vi "CRYSet Graph Property.vi"(4 "PreviewGraph Ref":refnum<vi>, 6 "Splitters":refnum<vi>[](array[refnum]), 7 "pGraph VI In":refnum<vi>, 8 "Panes":refnum<vi>[](array[refnum]), 9 "Graph Ref":refnum<vi>, 10 "Graph Type":string, 11 "Event Name":string) -> ()   [LabVIEW 2013]
uses:
  Control/CRYPolar Property.ctl
panel:
  in  "Polar Property":T1={"polar attributes"={"maximum"=2.0, "minimum"=0.0, "clip to min"=FALSE, "log"=FALSE, "grid color"=3381657, "plot color"=16711680, "fmt and prec"={"format"=enum."Decimal", "precision"=2}, "visible section"=4}, "Auto/Manual"=0, "Zero Adjust (deg)"=0, "Angle Increment (deg)"=0, "Mirror"=FALSE, "Auto Increment"=FALSE, "Total Rotatin (deg)"=0, "Discrete/Rannge"=0, "Show Name"=FALSE, "CurValues"=[], "CurIndex"=0, "CurColors"=[], "CurColors_Range"=[], "CurValues_Range"=[], "Pen"={"Width"=1, "Style"=enum."Solid"}, "BackgroundColor"=0} {"polar attributes"."minimum" format="%0.2f"; "polar attributes"."maximum" format="%0.2f"}
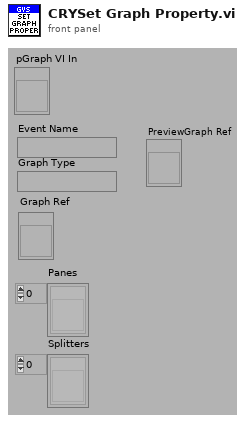
[diagram p1: front panel]
types:
  T1 = typedef "CRYPolar Property.ctl" = cluster{"polar attributes":cluster{"maximum":dbl, "minimum":dbl, "clip to min":bool, "log":bool, "grid color":u32, "plot color":u32, "fmt and prec":cluster{"format":enum8{"Decimal", "Scientific", "Engineering", "Binary", "Octal", "Hex"}, "precision":u8}, "visible section":u16}, "Auto/Manual":u16, "Zero Adjust (deg)":i32, "Angle Increment (deg)":i32, "Mirror":bool, "Auto Increment":bool, "Total Rotatin (deg)":i32, "Discrete/Rannge":u16, "Show Name":bool, "CurValues":dbl[], "CurIndex":u16, "CurColors":u32[], "CurColors_Range":u32[], "CurValues_Range":dbl[], "Pen":cluster{"Width":u16, "Style":enum32{"Solid", "Dash", "Dot", "DashDot", "DashDotDot"}}, "BackgroundColor":u32}
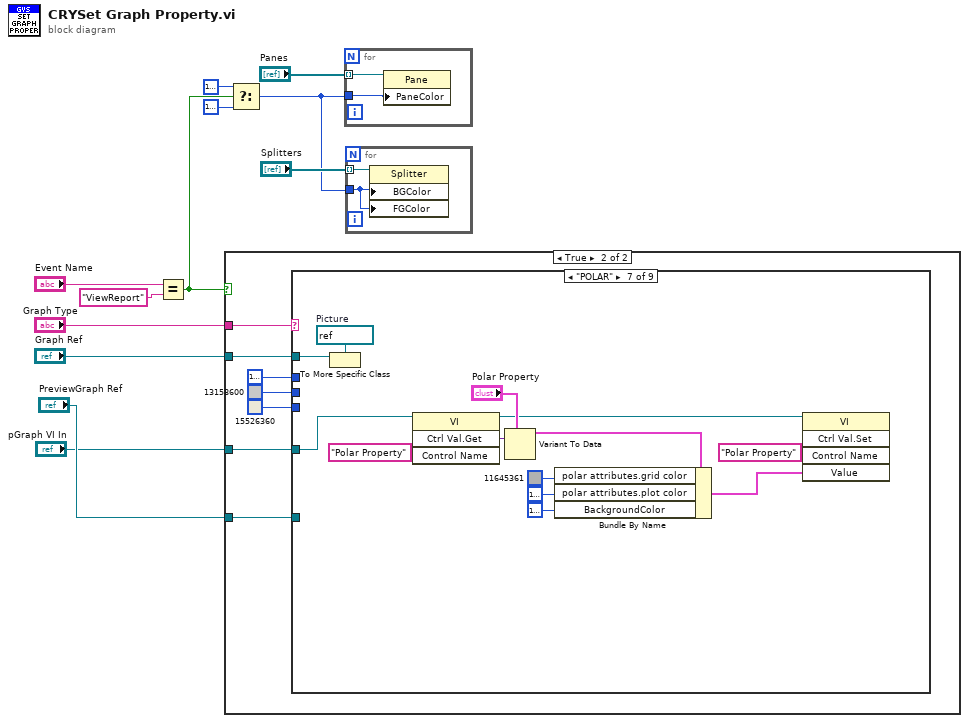
[diagram p0: block diagram]
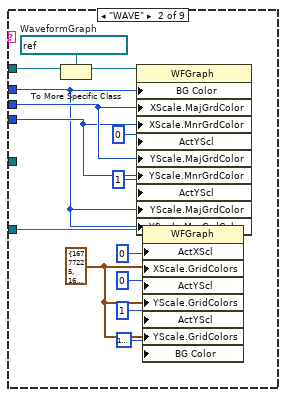
[diagram p4: hidden frame]
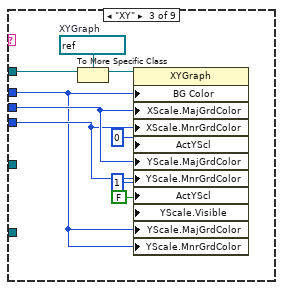
[diagram p5: hidden frame]
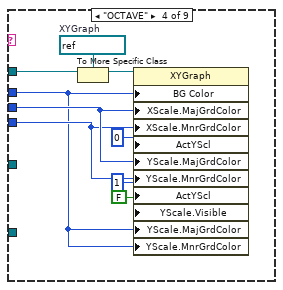
[diagram p6: hidden frame]
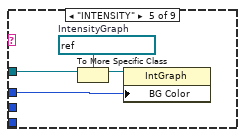
[diagram p7: hidden frame]
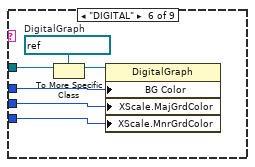
[diagram p8: hidden frame]
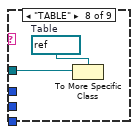
[diagram p9: hidden frame]
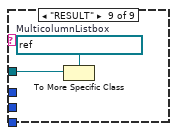
[diagram p10: hidden frame]
diagram:
  n1 = Equal?(x="Event Name", y="ViewReport" ("regular expression")) -> (x = y?=w5:bool)
  n2 = case shown="True" w5 {
    tunnel: "Graph Type" -> [_ w19]
    tunnel: "Graph Ref" -> [_ w18]
    tunnel: "PreviewGraph Ref" -> [_ w14]
    tunnel: "pGraph VI In" -> [_ w13]
    frame False {
    }
    frame True {
      n3 = case shown="\"POLAR\"" w19 {
        tunnel: w18 -> [_ w29 w38 w47 w55 w58 w74 w76 w78]
        tunnel: u32 16777226 -> [_ w26 w34 w43 w52 w61 _ _ _]
        tunnel: u32 13158600 -> [_ w31 w40 w49 _ w60 _ _ _]
        tunnel: u32 15526360 -> [_ w30 w39 w48 _ w59 _ _ _]
        tunnel: w14 -> [_ w22 _ _ _ _ _ _ _]
        tunnel: w13 -> [_ _ _ _ _ _ w69 _ _]
        frame Default {
        }
        frame "WAVE" {
          w23 = cluster{u32, u32} {16777225, 16777225}
          w27 = refnum<vi> refnum  # WaveformGraph
          n4 = To More Specific Class(target class=w27, reference=w29) -> (specific class reference=w28:refnum<vi>)  [unwired: 1 in, 1 out]
          n5 = property class="WFGraph"(reference=w28, "BG Color"=w26, "XScale.MajGrdColor"=w31, "XScale.MnrGrdColor"=w30, "ActYScl"=0 ("Active Y Scale"), "YScale.MajGrdColor"=w31, "YScale.MnrGrdColor"=w30, "ActYScl"=1 ("Active Y Scale"), "YScale.MajGrdColor"=w26, "YScale.MnrGrdColor"=w26) -> ()  [unwired: 1 in, 2 out]
          n6 = property on="Property Node" class="WFGraph"(reference=w22, "ActXScl"=0 ("Active X Scale"), "XScale.GridColors"=w23, "ActYScl"=0 ("Active Y Scale"), "YScale.GridColors"=w23, "ActYScl"=1 ("Active Y Scale"), "YScale.GridColors"=w23, "BG Color"=u32 16777225) -> ()  [unwired: 1 in, 2 out]
        }
        frame "XY" {
          w36 = refnum<vi> refnum  # XYGraph
          n7 = To More Specific Class(target class=w36, reference=w38) -> (specific class reference=w37:refnum<vi>)  [unwired: 1 in, 1 out]
          n8 = property class="XYGraph"(reference=w37, "BG Color"=w34, "XScale.MajGrdColor"=w40, "XScale.MnrGrdColor"=w39, "ActYScl"=0 ("Active Y Scale"), "YScale.MajGrdColor"=w40, "YScale.MnrGrdColor"=w39, "ActYScl"=1 ("Active Y Scale"), "YScale.Visible"=FALSE ("Y Scale.Visible"), "YScale.MajGrdColor"=w34, "YScale.MnrGrdColor"=w34) -> ()  [unwired: 1 in, 2 out]
        }
        frame "OCTAVE" {
          w45 = refnum<vi> refnum  # XYGraph
          n9 = To More Specific Class(target class=w45, reference=w47) -> (specific class reference=w46:refnum<vi>)  [unwired: 1 in, 1 out]
          n10 = property class="XYGraph"(reference=w46, "BG Color"=w43, "XScale.MajGrdColor"=w49, "XScale.MnrGrdColor"=w48, "ActYScl"=0 ("Active Y Scale"), "YScale.MajGrdColor"=w49, "YScale.MnrGrdColor"=w48, "ActYScl"=1 ("Active Y Scale"), "YScale.Visible"=FALSE ("Y Scale.Visible"), "YScale.MajGrdColor"=w43, "YScale.MnrGrdColor"=w43) -> ()  [unwired: 1 in, 2 out]
        }
        frame "INTENSITY" {
          w53 = refnum<vi> refnum  # IntensityGraph
          n11 = To More Specific Class(target class=w53, reference=w55) -> (specific class reference=w54:refnum<vi>)  [unwired: 1 in, 1 out]
          n12 = property class="IntGraph"(reference=w54, "BG Color"=w52) -> ()  [unwired: 1 in, 2 out]
        }
        frame "DIGITAL" {
          w56 = refnum<vi> refnum  # DigitalGraph
          n13 = To More Specific Class(target class=w56, reference=w58) -> (specific class reference=w57:refnum<vi>)  [unwired: 1 in, 1 out]
          n14 = property class="DigitalGraph"(reference=w57, "BG Color"=w61, "XScale.MajGrdColor"=w60, "XScale.MnrGrdColor"=w59) -> ()  [unwired: 1 in, 2 out]
        }
        frame "POLAR" {
          w73 = refnum<vi> refnum  # Picture
          n15 = To More Specific Class(target class=w73, reference=w74) -> ()  [unwired: 1 in, 2 out]
          n16 = invoke class="VI" method="Ctrl Val.Get"(reference=w69, "Control Name"="Polar Property") -> (reference out=w67:refnum<vi>, "Get Control Value Variant"=w71:variant)  [unwired: 2 in, 2 out]
          n17 = Variant To Data(type="Polar Property", Variant=w71) -> (data=w66:T1)  [unwired: 1 in, 1 out]
          n18 = Bundle By Name(cluster=w66, "polar attributes.grid color"=u32 11645361 ("grid color"), "polar attributes.plot color"=u32 16777222, "BackgroundColor"=u32 16777226) -> (w65:T1)
          n19 = invoke class="VI" method="Ctrl Val.Set"(reference=w67, "Control Name"="Polar Property", "Value"=w65) -> ()  [unwired: 2 in, 5 out]
        }
        frame "TABLE" {
          w75 = refnum<vi> refnum  # Table
          n20 = To More Specific Class(target class=w75, reference=w76) -> ()  [unwired: 1 in, 2 out]
        }
        frame "RESULT" {
          w77 = refnum<vi> refnum  # MulticolumnListbox
          n21 = To More Specific Class(target class=w77, reference=w78) -> ()  [unwired: 1 in, 2 out]
        }
      }
    }
  }
  n22 = Select(t=u32 16777226, s=w5, f=u32 16777238) -> (s? t:f=w3:u32)
  n23 = for {
    tunnel: "Panes" -> [w80] mode=indexing
    tunnel: w3 -> [w79]
    n24 = property class="Pane"(reference=w80, "PaneColor"=w79) -> ()  [unwired: 1 in, 2 out]
  }
  n25 = for {
    tunnel: "Splitters" -> [w82] mode=indexing
    tunnel: w3 -> [w81]
    n26 = property class="Splitter"(reference=w82, "BGColor"=w81, "FGColor"=w81) -> ()  [unwired: 1 in, 2 out]
  }
